vi "FindSymbolInDir.vi"(8 "error in (no error)":errorcluster, 10 "pattern":string="开发环境 *", 11 "path":path) -> (0 "error out":errorcluster, 1 "String":string, 2 "Exits?":bool, 3 "path (dup)":path)   [LabVIEW 2017, in "application.lvlib" / "application.lvclass"]
uses:
  application.lvclass
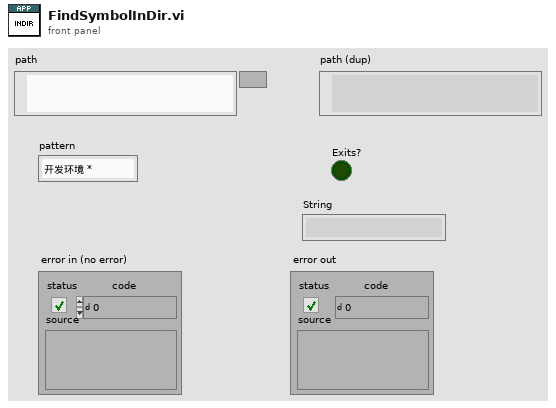
[diagram p1: front panel]
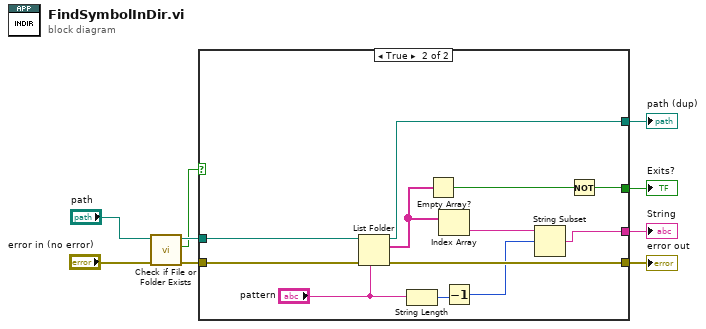
[diagram p0: block diagram]
diagram:
  n1 = call <vilib>:"Check if File or Folder Exists.vi"("error in (no error)"="error in (no error)", "path"="path") -> ("error out"=w6:errorcluster, "file or folder exists?"=w5:bool, "dup path"=w7:path)  [unwired: 7 in]
  n2 = case shown="True" w5 {
    tunnel: w7 -> [w10 w19]
    tunnel: w6 -> [w11 w23]
    tunnel: [w11 w17] -> w8
    tunnel: [_ w21] -> w3
    tunnel: [_ w12] -> w2
    tunnel: [w10 w20] -> w1
    frame False {
    }
    frame True {
      n3 = List Folder(path=w19, pattern="pattern", error in=w23) -> (path out=w20:path, filenames=w18:string[], error out=w17:errorcluster)  [unwired: 1 in, 1 out]
      n4 = String Length(string="pattern") -> (length=w14:i32)
      n5 = Empty Array?(array=w18) -> (empty?=w22:bool)
      n6 = Index Array(array=w18) -> (element=w16:string)  [unwired: 1 in]
      n7 = Decrement(x=w14) -> (x-1=w13:i32)
      n8 = String Subset(string=w16, offset (0)=w13) -> (substring=w12:string)  [unwired: 1 in]
      n9 = Not(x=w22) -> (.not. x?=w21:bool)
    }
  }
  "error out" <- w8
  "Exits?" <- w3
  "String" <- w2
  "path (dup)" <- w1
